vi "Device Connection Test App.vi"() -> ()   [LabVIEW 2011]
uses:
  Private/Type Defs/Interface.ctl
  LVH-LINX.lvlib
panel:
  out "Error Out":errorcluster
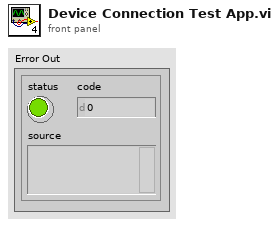
[diagram p1: front panel]
types:
  T1 = typedef "LVH-LINX.lvlib/Interface.ctl" = enum16{"Serial", "TCP"}
  T2 = typedef "LVH-LINX.lvlib/LINX Device Config.ctl" = cluster{"Interface":T1, "COM Port":refnum<visa-resource-name>, "Packet Number":u16, "TCP Configuration":T3}
  T3 = typedef "LVH-LINX.lvlib/TCP Config.ctl" = cluster{"IP Address":string, "Port":dbl}
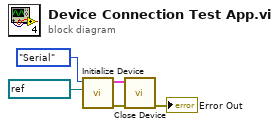
[diagram p0: block diagram]
diagram:
  n1 = call "Initialize Device.vi"("COM Port"=refnum<visa-resource-name> "COM5", "Interface"=Interface."Serial") -> ("Error Out"=w1:errorcluster, "LINX Device Config"=w2:T2)  [unwired: 8 in]
  n2 = call "Close Device.vi"("Error In"=w1, "LINX Device Config"=w2) -> ("Error Out"=→"Error Out":errorcluster)  [unwired: 9 in]
